vi "Commit.vi"(6 "All":bool, 8 "error in (no error)":errorcluster, 9 "Files to Add":path[](array[path]), 10 "Message":string, 11 "Git Implementation in":refnum<class "Git Implementation.lvclass">) -> (0 "error out":errorcluster, 2 "Status Message":string, 3 "Git Implementation out":refnum<class "Git Implementation.lvclass">)   [LabVIEW 2017, in "Git-LabVIEW.lvlib" / "Git Implementation.lvclass"]
doc: "Create a new commit containing the current contents of the index."
uses:
  Git Implementation.lvclass
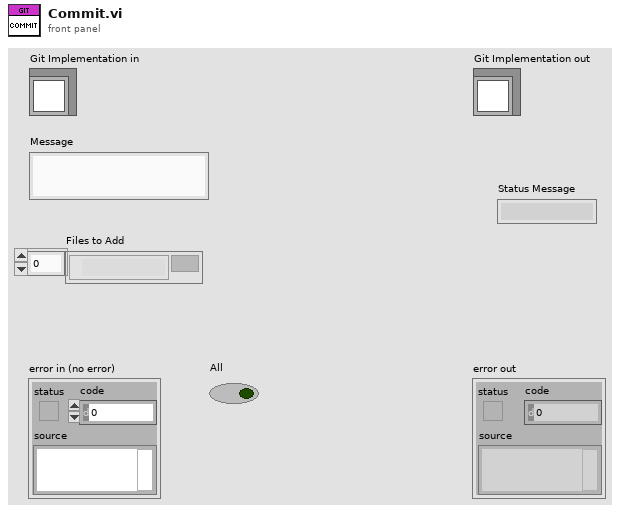
[diagram p1: front panel]
types:
  T1 = typedef "Git-LabVIEW.lvlib/Git Implementation.lvclass/CMD Return.ctl" = cluster{"StdOut":string, "StdErr":string, "Return Code":i32}
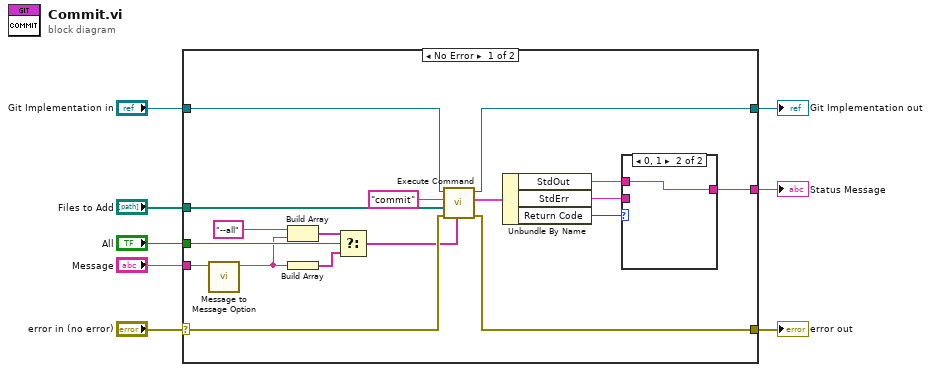
[diagram p0: block diagram]
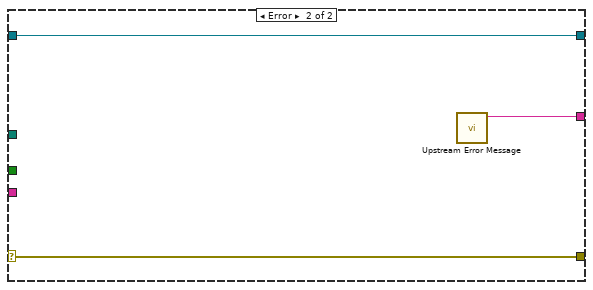
[diagram p3: hidden frame]
diagram:
  n1 = case shown="No Error" "error in (no error)" {
    selector: "error in (no error)" -> [w26 w31]
    tunnel: [w25 w31] -> w7
    tunnel: [w21 w30] -> w5
    tunnel: "Git Implementation in" -> [w22 w30]
    tunnel: "Message" -> [w20 _]
    tunnel: "Files to Add" -> [w24 _]
    tunnel: "All" -> [w19 _]
    tunnel: [w11 w29] -> w1
    frame No Error {
      n2 = call "Message to Message Option.vi"("Message"=w20) -> ("Message Option"=w16:string)  [unwired: 10 in]
      n3 = Build Array("--all" ("element"), w16) -> (w17:string[])
      n4 = Build Array(w16) -> (w18:string[])
      n5 = Select(t=w17, s=w19, f=w18) -> (s? t:f=w14:string[])
      n6 = call "Execute Command.vi"("Arguments"=w14, "error in (no error)"=w26, "File Paths"=w24, "Command"="commit", "Git Implementation in"=w22) -> ("error out"=w25:errorcluster, "CMD Return"=w13:T1, "Git Implementation out"=w21:refnum<class "Git Implementation.lvclass">)  [unwired: 4 in]
      n7 = Unbundle By Name(w13) -> ("StdOut"=w9:string, "StdErr"=w10:string, "Return Code"=w12:i32)
      n8 = case shown="0, 1" w12 {
        tunnel: [w27 w28] -> w11
        tunnel: w10 -> [w27 _]
        tunnel: w9 -> [_ w28]
        frame Default {
        }
        frame 0, 1 {
        }
      }
    }
    frame Error {
      n9 = call "Upstream Error Message.vi"() -> ("Upstream Error Message"=w29:string)  [unwired: 11 in]
    }
  }
  "error out" <- w7
  "Git Implementation out" <- w5
  "Status Message" <- w1
